vi "Track Best Ball.vi"(8 "Tracking mode":T4, 9 "Ball Camera Type":T1, 10 "Camera Image":T3, 11 "Ranked Balls":T5(array[cluster]) {"Score" format="%#.1g"}) -> (3 "Ball Track Cluster":T2)   [LabVIEW 2015]
uses:
  Common Code/Tracking Mode.ctl
  <vilib>/vision/Image Controls.llb/IMAQ Image.ctl
  Common Code/Ball Tracking Command Cluster.ctl
  Camera Types.ctl
panel:
  in  "Ball Camera Type 2":T1
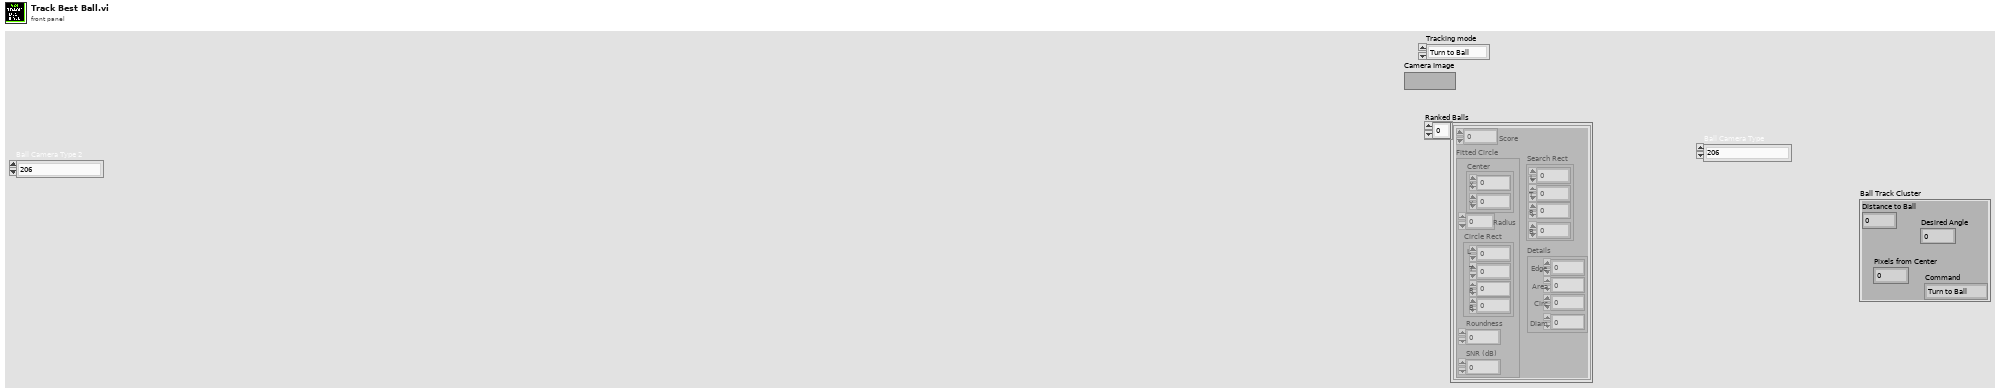
[diagram p1: front panel]
types:
  T1 = typedef "Camera Types.ctl" = enum16{"206", "1011", "1013", "MS HD3000 square", "MS HD3000 640x480"}
  T2 = typedef "Ball Tracking Command Cluster.ctl" = cluster{"Distance to Ball":dbl, "Desired Angle":dbl, "Command":enum16{"Turn to Ball", "Turn to Angle", "Get Distance"}, "Pixels from Center":dbl}
  T3 = typedef "IMAQ Image.ctl" = refnum<image>
  T4 = typedef "Tracking Mode.ctl" = enum16{"Turn to Ball", "Turn to Angle"}
  T5 = cluster{"Score":sgl, "Fitted Circle":cluster{"Center":cluster{"X":sgl, "Y":sgl}, "Radius":dbl, "Circle Rect":cluster{"L":sgl, "T":sgl, "R":sgl, "B":sgl}, "Roundness":dbl, "SNR (dB)":dbl}, "Search Rect":cluster{"L":sgl, "T":sgl, "R":sgl, "B":sgl}, "Details":cluster{"Edge":sgl, "Area":sgl, "Circ":sgl, "Diam":sgl}}[]
  T6 = typedef "Image Type" = u32
  T7 = cluster{"Score":sgl, "Fitted Circle":cluster{"Center":cluster{"X":sgl, "Y":sgl}, "Radius":dbl, "Circle Rect":cluster{"L":sgl, "T":sgl, "R":sgl, "B":sgl}, "Roundness":dbl, "SNR (dB)":dbl}, "Search Rect":cluster{"L":sgl, "T":sgl, "R":sgl, "B":sgl}, "Details":cluster{"Edge":sgl, "Area":sgl, "Circ":sgl, "Diam":sgl}}
  T8 = cluster{"Center":cluster{"X":sgl, "Y":sgl}, "Radius":dbl, "Circle Rect":cluster{"L":sgl, "T":sgl, "R":sgl, "B":sgl}, "Roundness":dbl, "SNR (dB)":dbl}
  T9 = cluster{"Edge":sgl, "Area":sgl, "Circ":sgl, "Diam":sgl}
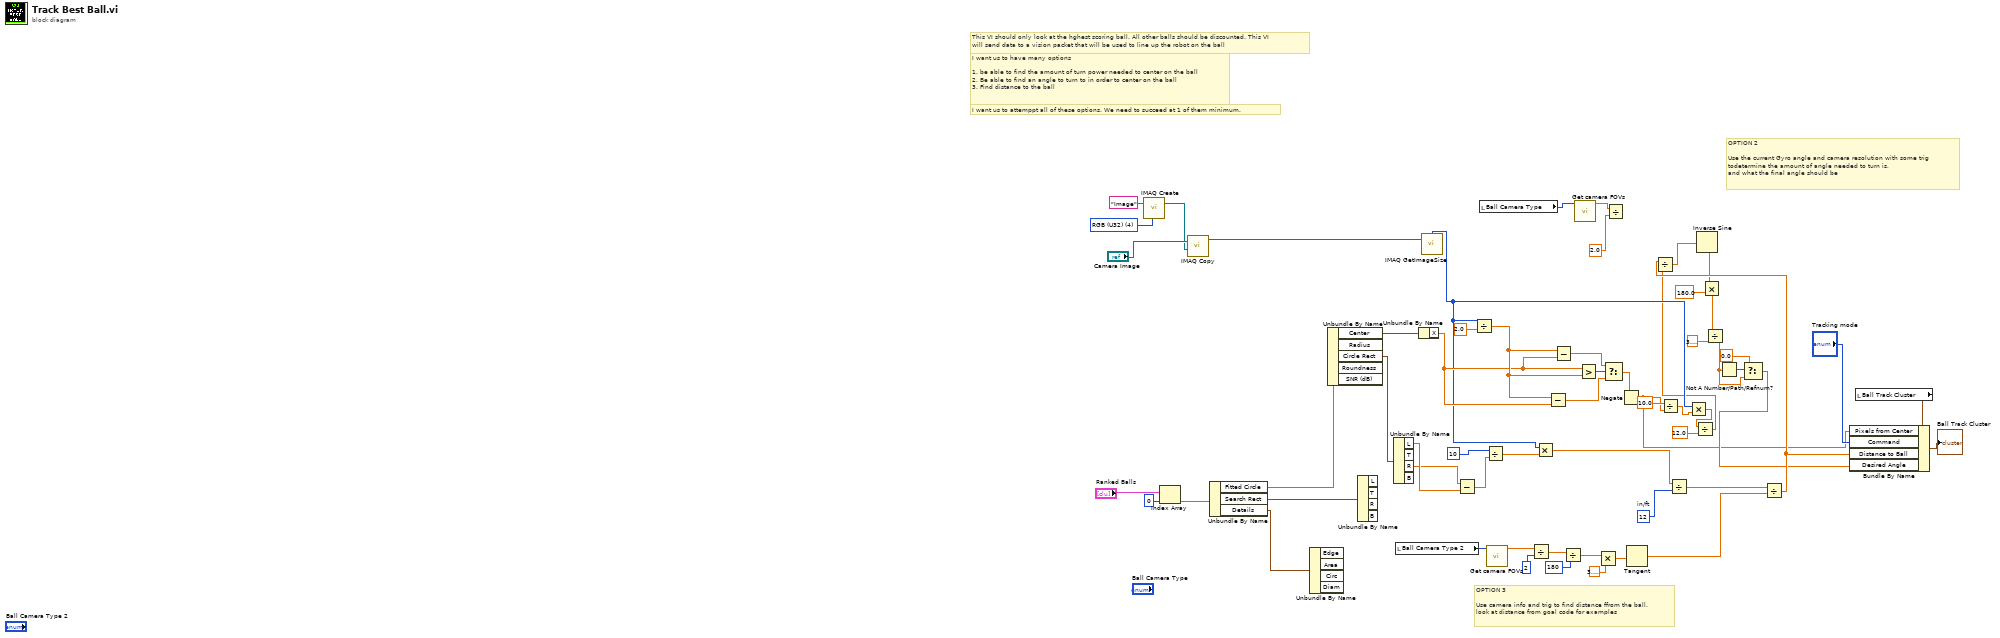
[diagram p0: block diagram]
diagram:
  w38 = 12  # in/ft
  w50 = T6 4 items=["Grayscale (U8)", "Grayscale (I16)", "Grayscale (SGL)", "Complex (CSG)", "RGB (U32)", "HSL (U32)", "RGB (U64)", "Grayscale (U16)"] ("Image Type")
  # "OPTION 3\n\nUse camera info and trig to find distance ffrom the ball.\nlook at distance from goal code for examples"
  # "This VI should only look at the hghest scoring ball. All other balls should be discounted. This VI\nwill send data to a vision packet that will be used to line up the robot on the ball"
  # "I want us to attemppt all of these options. We need to succeed at 1 of them minimum."
  # "OPTION 2\n\nUse the current Gyro angle and camera resolution with some trig\ntodetermine the amount of angle needed to turn is, \nand what the final angle should be"
  # "I want us to have many options\n\n1. be able to find the amount of turn power needed to center on the ball\n2. Be able to find an angle to turn to in order to center on the ball\n3. Find distance to the ball"
  n1 = call "IMAQ Create"("Image Name"="Image", "Image Type"=w50) -> ("New Image"=w53:T3)  [unwired: 3 in, 1 out]
  n2 = Index Array(array="Ranked Balls", index=0) -> (element=w58:T7)
  n3 = call "IMAQ Copy"("Image Dst"=w53, "Image Src"="Camera Image") -> ("Image Dst Out"=w52:T3)  [unwired: 4 in, 1 out]
  n4 = Unbundle By Name(w58) -> ("Fitted Circle"=w55:T8, "Search Rect"=w56:cluster{"L":sgl, "T":sgl, "R":sgl, "B":sgl}, "Details"=w57:T9)
  n5 = Unbundle By Name(w57) -> ()  [unwired: 4 out]
  n6 = Unbundle By Name(w55) -> ("Center"=w27:cluster{"X":sgl, "Y":sgl}, "Circle Rect"=w26:cluster{"L":sgl, "T":sgl, "R":sgl, "B":sgl})  [unwired: 3 out]
  n7 = Unbundle By Name(w56) -> ()  [unwired: 4 out]
  n8 = Unbundle By Name(w26) -> ("L"=w25:sgl, "R"=w24:sgl)  [unwired: 2 out]
  n9 = local read "Ball Camera Type 2"() -> (w32:T1)
  n10 = Unbundle By Name(w27) -> ("X"=w17:sgl)
  n11 = call "IMAQ GetImageSize"("Image"=w52) -> ("X Resolution"=w5:i32)  [unwired: 3 in, 2 out]
  n12 = Subtract(x=w24, y=w25) -> (x-y=w40:sgl)
  n13 = Divide(x=w5, y=2.0) -> (x/y=w47:dbl)
  n14 = local read "Ball Camera Type"() -> (w23:T1)
  n15 = Divide(x=10, y=w40) -> (x/y=w41:sgl)
  n16 = call "Get camera FOVs.vi"("Camera Type"=w32) -> ("FOV"=w33:dbl)  [unwired: 9 in, 1 out]
  n17 = Divide(x=w33, y=2) -> (x/y=w34:dbl)
  n18 = Multiply(x=w5, y=w41) -> (x*y=w42:sgl)
  n19 = Subtract(x=w47, y=w17) -> (x-y=w46:dbl)
  n20 = Subtract(x=w47, y=w17) -> (x-y=w13:dbl)
  n21 = Divide(x=w34, y=180) -> (x/y=w35:dbl)
  n22 = call "Get camera FOVs.vi"("Camera Type"=w23) -> ("FOV"=w21:dbl)  [unwired: 9 in, 1 out]
  n23 = Greater?(x=w17, y=w47) -> (0:w44:bool)
  n24 = Multiply(x=w35, y=3.141592653589793) -> (x*y=w36:dbl)
  n25 = Select(t=w13, s=w44, f=w46) -> (s? t:f=w12:dbl)
  n26 = Divide(x=w21, y=2.0) -> ()  [unwired: 1 out]
  n27 = Negate(x=w12) -> (-x=w1:dbl)
  n28 = Tangent(1:w36) -> (0:w37:dbl)
  n29 = Divide(x=10.0, y=w1) -> (x/y=w6:dbl)
  n30 = Divide(x=w42, y=w38) -> (x/y=w43:sgl)
  n31 = Multiply(x=w5, y=w6) -> (x*y=w4:dbl)
  n32 = Divide(x=w4, y=12.0) -> (x/y=w3:dbl)
  n33 = Divide(x=w43, y=w37) -> (x/y=w20:dbl)
  n34 = Divide(x=w20, y=w3) -> (x/y=w19:dbl)
  n35 = Inverse Sine(1:w19) -> (0:w18:dbl)
  n36 = Multiply(x=w18, y=180.0) -> (x*y=w16:dbl)
  n37 = Divide(x=w16, y=3.141592653589793) -> (x/y=w9:dbl)
  n38 = Not A Number/Path/Refnum?(number/path/refnum=w9) -> (NaN/Path/Refnum?=w11:bool)
  n39 = Select(t=0.0, s=w11, f=w9) -> (s? t:f=w8:dbl)
  n40 = local read "Ball Track Cluster"() -> (w48:T2)
  n41 = Bundle By Name(cluster=w48, "Pixels from Center"=w1, "Command"="Tracking mode", "Distance to Ball"=w20, "Desired Angle"=w8) -> (→"Ball Track Cluster":T2)
